vi "FTW-ActorExtended-Subscription-Remove.vi"(0 "FTW-ActorExtended In":refnum<class "FTW-ActorExtended.lvclass">, 5 "Subscriber Name":string, 11 "error in":errorcluster) -> (4 "FTW-ActorExtended Out":refnum<class "FTW-ActorExtended.lvclass">, 15 "error out":errorcluster)   [LabVIEW 2015, in "FTW-ActorExtended.lvclass"]
uses:
  FTW-ActorExtended.lvclass
  FTW-ActorExtended.lvclass/FTW-ActorExtended.ctl
  Subscriber/FTW-Subscriber.lvclass
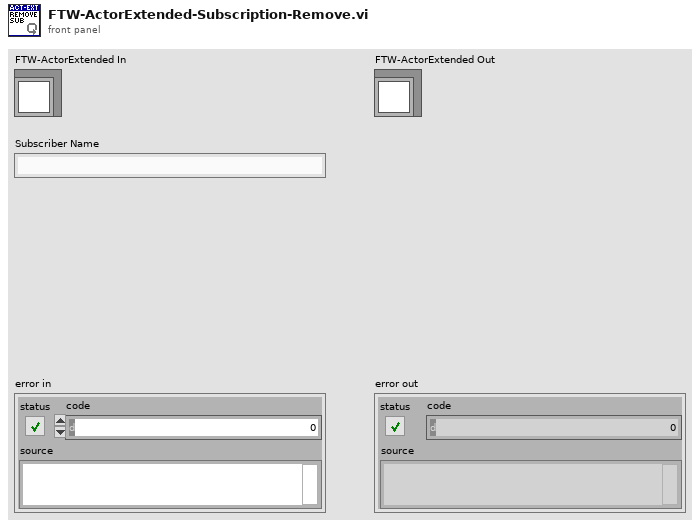
[diagram p1: front panel]
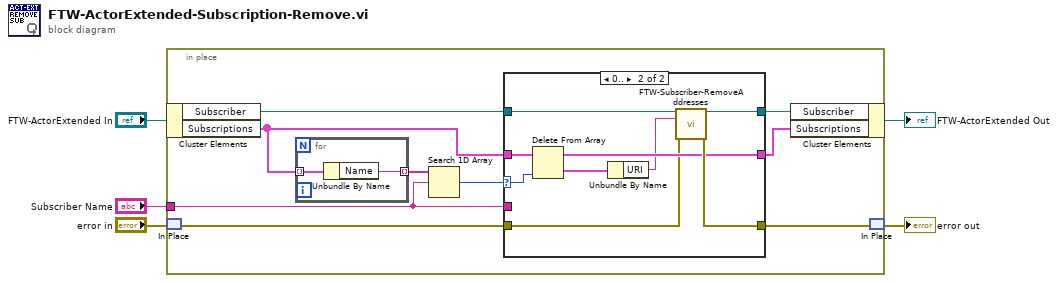
[diagram p0: block diagram]
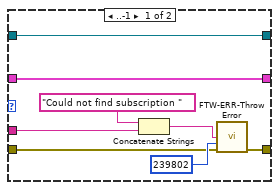
[diagram p2: hidden frame]
diagram:
  n1 = in-place {
    in-place-border: "Subscriber Name" -> [w7]
    n2 = in-place-cluster #1("FTW-ActorExtended In") -> ("Subscriber"=w14:refnum<class "FTW-Subscriber.lvclass">, "Subscriptions"=w10:cluster{"Name":string, "URI":string}[])
    n3 = in-place-match #2("error in") -> (w13:errorcluster)
    n4 = for {
      tunnel: w10 -> [w16] mode=indexing
      tunnel: [w15] -> w6 mode=indexing
      n5 = Unbundle By Name(w16) -> ("Name"=w15:string)
    }
    n6 = Search 1D Array(1D array=w6, element=w7) -> (index of element=w8:i32)  [unwired: 1 in]
    n7 = case shown="0.." w8 {
      selector: w8 -> [_ w28]
      tunnel: w14 -> [w24 w33]
      tunnel: w13 -> [w18 w27]
      tunnel: [w24 w32] -> w12
      tunnel: [w19 w31] -> w11
      tunnel: w10 -> [w23 w30]
      tunnel: [w23 w29] -> w9
      tunnel: w7 -> [w17 _]
      frame ..-1 {
        n8 = Concatenate Strings("Could not find subscription " ("string"), w17) -> (w22:string)
        n9 = call "FTW-ERR-ThrowError.vi"("Error Message"=w22, "Error Code"=239802, "error in"=w18) -> ("error out"=w19:errorcluster)  [unwired: 12 in]
      }
      frame 0.. {
        n10 = Delete From Array(array=w30, index=w28) -> (deleted portion=w26:cluster{"Name":string, "URI":string}, array with subset deleted=w29:cluster{"Name":string, "URI":string}[])  [unwired: 1 in]
        n11 = Unbundle By Name(w26) -> ("URI"=w25:string)
        n12 = call "FTW-Subscriber-RemoveAddresses.vi"("FTW-Subscription In"=w33, "Addresses"=w25, "error in"=w27) -> ("FTW-Subscription Out"=w32:refnum<class "FTW-Subscriber.lvclass">, "error out"=w31:errorcluster)  [unwired: 11 in]
      }
    }
    n13 = in-place-cluster #1("Subscriber"=w12, "Subscriptions"=w9) -> (→"FTW-ActorExtended Out":refnum<class "FTW-ActorExtended.lvclass">)
    n14 = in-place-match #2(w11) -> (→"error out":errorcluster)
  }
